vi "未命名 1.vi"() -> ()   [LabVIEW 2016, in "自动更新.lvlib"]
panel:
  in  "更新":bool
  in  "updateconfiguration":T1={"主机"="27.154.58.30", "用户"="update", "密码"="std23506", "远程路径"="数据传输系统\\平台数据传输系统.exe", "下载文件名"="平台数据传输系统.exe", "软件版本"=""}
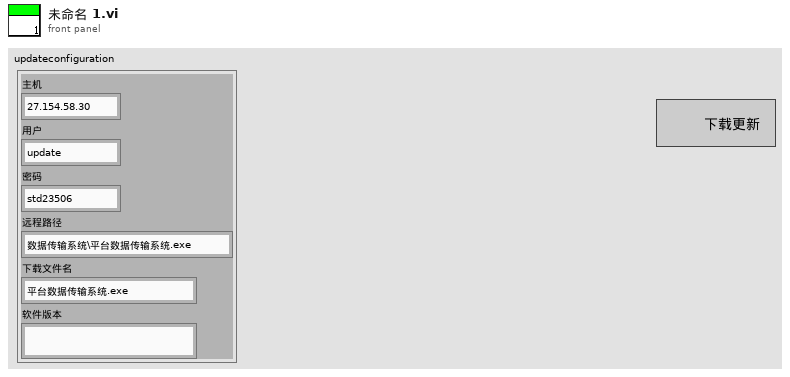
[diagram p1: front panel]
types:
  T1 = cluster{"主机":string, "用户":string, "密码":string, "远程路径":string, "下载文件名":string, "软件版本":string}
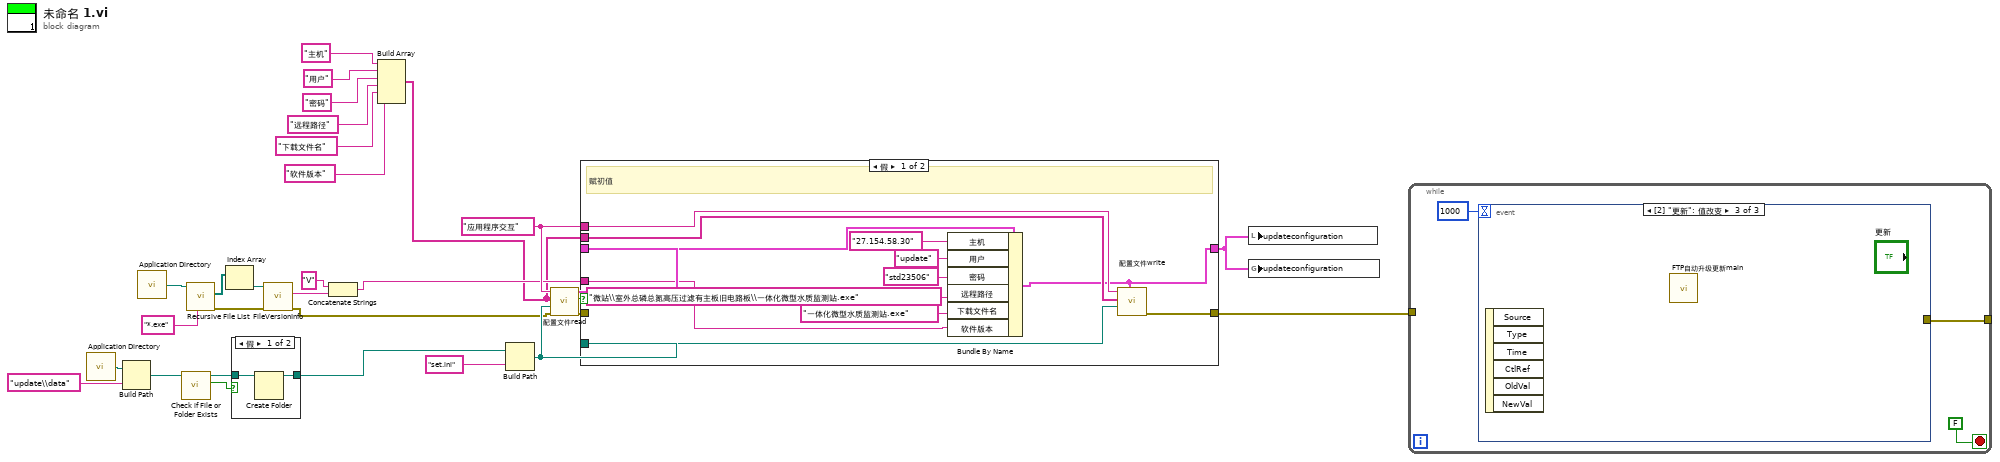
[diagram p0: block diagram]
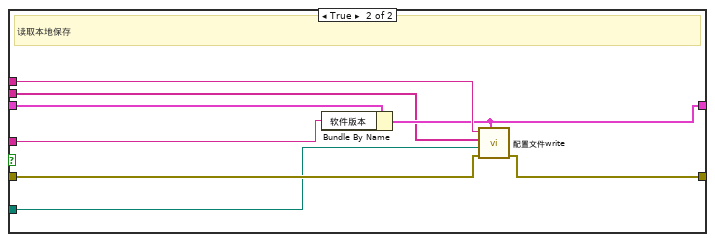
[diagram p3: hidden frame]
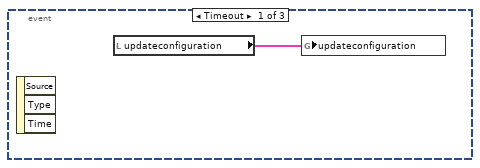
[diagram p4: hidden frame]
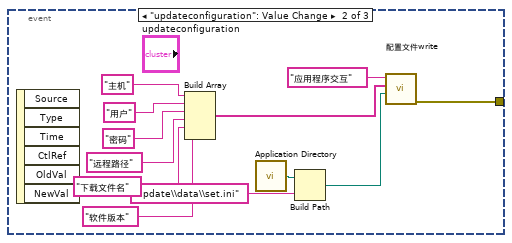
[diagram p5: hidden frame]
diagram:
  w28 = "应用程序交互" ("section")
  n1 = call <vilib>:"Application Directory.vi"() -> ("Application Directory"=w5:path)
  n2 = Build Path(base path=w5, name or relative path="update\\data" ("名称或相对路径")) -> (appended path=w6:path)
  n3 = call <vilib>:"Application Directory.vi"() -> ("Application Directory"=w23:path)
  n4 = call <vilib>:"Check if File or Folder Exists.vi"("path"=w6) -> ("file or folder exists?"=w7:bool, "dup path"=w8:path)  [unwired: 8 in, 1 out]
  n5 = call <vilib>:"Recursive File List.vi"("pattern"="*.exe", "Folder Path"=w23) -> ("error out"=w20:errorcluster, "All Files in Dir"=w22:path[])  [unwired: 5 in, 3 out]
  n6 = Index Array(array=w22) -> (element=w24:path)  [unwired: 1 in]
  n7 = case shown="假" w7 {
    tunnel: w8 -> [w32 w33]
    tunnel: [w31 w33] -> w3
    frame False {
      n8 = Create Folder(path (use dialog)=w32) -> (created path=w31:path)  [unwired: 2 in, 2 out]
    }
    frame True {
    }
  }
  n9 = call <vilib>:"FileVersionInfo.vi"("error in (no error)"=w20, "Application Path in"=w24) -> ("error out"=w17:errorcluster, "File Version Info"=w18:string)  [unwired: 6 in, 2 out]
  n10 = Concatenate Strings("V" ("字符串"), w18) -> (w16:string)
  n11 = Build Array("主机" ("section"), "用户" ("section"), "密码" ("key"), "远程路径" ("key"), "下载文件名" ("key"), "软件版本" ("key")) -> (w2:string[])
  n12 = Build Path(base path=w3, name or relative path="set.ini" ("名称或相对路径")) -> (appended path=w27:path)
  n13 = call "配置文件read.vi"("error in (no error)"=w17, "configuration file path"=w27, "键数组"=w2, "段"=w28) -> ("error out"=w26:errorcluster, "section exists?"=w29:bool, "updateconfiguration"=w25:T1)  [unwired: 5 in]
  n14 = case shown="假" w29 {
    tunnel: w2 -> [w45 w49]
    tunnel: w28 -> [w44 w53]
    tunnel: w27 -> [w43 w47]
    tunnel: w26 -> [_ w48]
    tunnel: [w42 w46] -> w15
    tunnel: w25 -> [w36 w52]
    tunnel: [w34 w50] -> w1
    tunnel: w16 -> [w35 w51]
    frame False {
      # "赋初值"
      n15 = Bundle By Name(cluster=w36, "主机"="27.154.58.30" ("key"), "用户"="update", "密码"="std23506", "远程路径"="微站\\室外总磷总氮高压过滤有主板旧电路板\\一体化微型水质监测站.exe", "下载文件名"="一体化微型水质监测站.exe", "软件版本"=w35) -> (w34:T1)
      n16 = call "配置文件write.vi"("updateconfiguration"=w34, "configuration file path"=w43, "键数组"=w45, "段"=w44) -> ("error out"=w42:errorcluster)  [unwired: 7 in]
    }
    frame True {
      # "读取本地保存"
      n17 = Bundle By Name(cluster=w52, "软件版本"=w51) -> (w50:T1)
      n18 = call "配置文件write.vi"("updateconfiguration"=w50, "error in (no error)"=w48, "configuration file path"=w47, "键数组"=w49, "段"=w53) -> ("error out"=w46:errorcluster)  [unwired: 6 in]
    }
  }
  n19 = local write "updateconfiguration"(w1) -> ()
  n20 = global write "update全局.vi" "updateconfiguration"(w1) -> ()
  n21 = while {
    tunnel: [w54] -> _
    tunnel: w15 -> [_]
    stop <- FALSE stop-if-true
    n22 = event shown="[2] \"更新\": 值改变" {
      selector: _ -> [_ _ _]
      dyn-events: _ -> [_ _ _]
      timeout: 1000 -> [_ _ _]
      tunnel: [_ w65 _] -> w54
      event Timeout {
        n23 = event-data() -> ()  [unwired: 1 in, 3 out]
        n24 = local read "updateconfiguration"() -> (w57:T1)
        n25 = global write "update全局.vi" "updateconfiguration"(w57) -> ()
      }
      event "updateconfiguration": Value Change {
        n26 = event-data() -> ()  [unwired: 1 in, 6 out]
        n27 = Build Array("主机" ("section"), "用户" ("section"), "密码" ("key"), "远程路径" ("key"), "下载文件名" ("key"), "软件版本" ("key")) -> (w58:string[])
        n28 = call <vilib>:"Application Directory.vi"() -> ("Application Directory"=w68:path)
        n29 = Build Path(base path=w68, name or relative path="update\\data\\set.ini" ("名称或相对路径")) -> (appended path=w66:path)
        n30 = call "配置文件write.vi"("configuration file path"=w66, "键数组"=w58, "段"="应用程序交互" ("section")) -> ("error out"=w65:errorcluster)  [unwired: 8 in]
      }
      event "更新": Value Change {
        n31 = event-data() -> ()  [unwired: 1 in, 6 out]
        n32 = call "FTP自动升级更新main.vi"() -> ()  [unwired: 12 in]
      }
    }
  }
